vi "MultiColumnListbox_UnColorRows.vi"(7 "Parent VI Reference":refnum<vi>, 8 "error in":errorcluster, 10 "Color Rows":u32(colorbox)=16448250, 11 "MCL Reference":refnum<vi>) -> (0 "error out":errorcluster)   [LabVIEW 2014, in "hse-ui.lvlib"]
doc: "Colors the rows of a MCLB in alternate colors. If <b>Parent VI Reference</b> is supplied, panel updates are deferred.\n\n____\nHAMPEL SOFTWARE ENGINEERING v0.7.0 (2018-07-16 18:12)"
uses:
  hse-ui.lvlib
  MulticolumnListControl__System.ctl
  <vilib>/Utility/miscctls.llb/LVRowAndColumnTypeDef.ctl
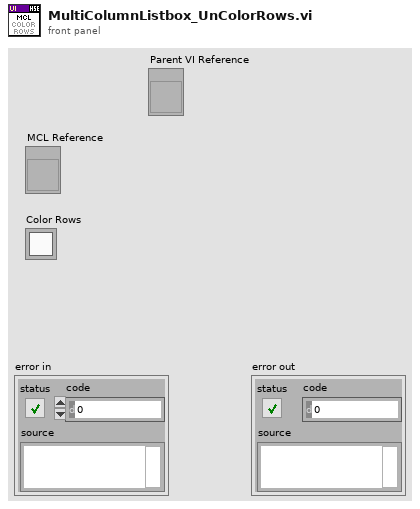
[diagram p1: front panel]
types:
  T1 = typedef "LVRowAndColumnTypeDef.ctl" = cluster{"Row":i32, "Column":i32}
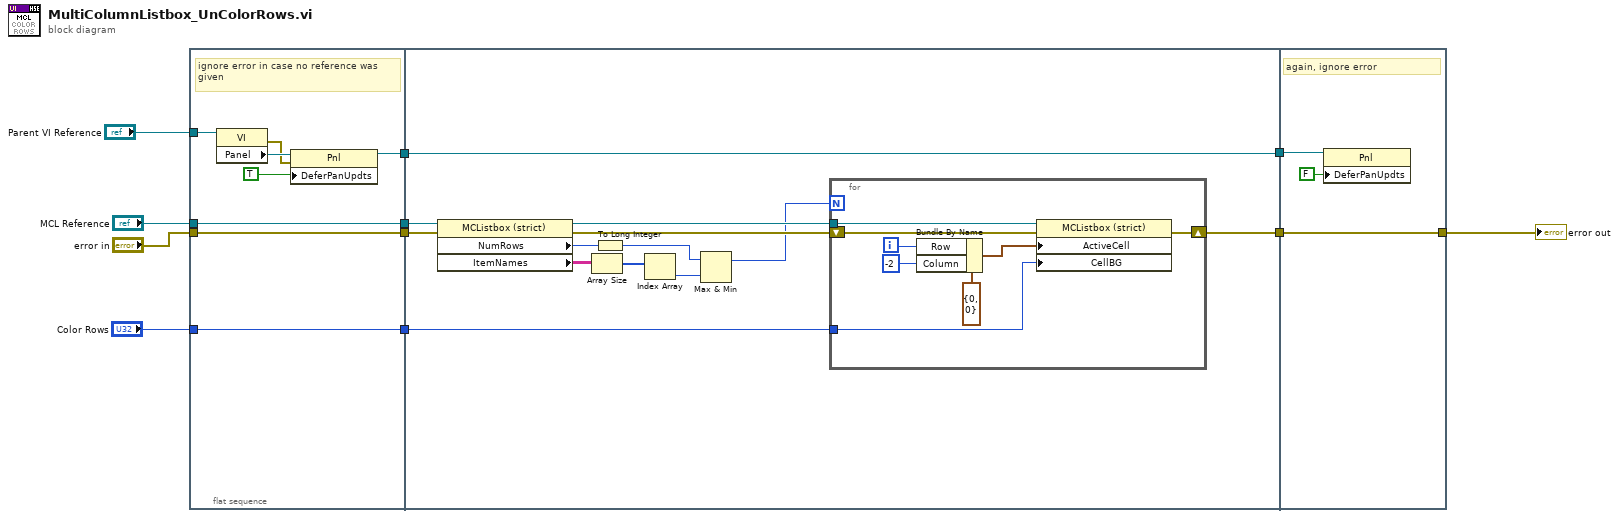
[diagram p0: block diagram]
diagram:
  n1 = flat-sequence {
    tunnel: "MCL Reference" -> [w19]
    tunnel: [w19] -> w10
    tunnel: [w15] -> w9
    tunnel: "error in" -> [w15]
    tunnel: "Parent VI Reference" -> [w14]
    tunnel: [w13] -> w6
    tunnel: "Color Rows" -> [w12]
    tunnel: [w12] -> w1
    tunnel: w10 -> [w26]
    tunnel: w9 -> [w24]
    tunnel: w6 -> [w23]
    tunnel: [w25] -> w5
    tunnel: [w23] -> w4
    tunnel: w1 -> [w21]
    tunnel: [w43] -> w3
    tunnel: w5 -> [w43]
    tunnel: w4 -> [w41]
    frame #0 {
      # "ignore error in case no reference was given"
      n2 = property class="VI"(reference=w14) -> (error out=w17:errorcluster, "Panel"=w18:refnum<vi>)  [unwired: 1 in, 1 out]
      n3 = property class="Pnl"(reference=w18, error in=w17, "DeferPanUpdts"=TRUE ("Defer Panel Updates")) -> (reference out=w13:refnum<vi>)  [unwired: 1 out]
    }
    frame #1 {
      n4 = property on="Property Node" class="MCListbox (strict)"(reference=w26, error in=w24) -> (reference out=w28:refnum<vi>, error out=w27:errorcluster, "NumRows"=w29:u32, "ItemNames"=w30:string[][])
      n5 = Array Size(array=w30) -> (size(s)=w32:i32[])
      n6 = To Long Integer(number=w29) -> (32bit integer=w22:i32)
      n7 = Index Array(array=w32) -> (element=w31:i32)  [unwired: 1 in]
      n8 = Max & Min(x=w22, y=w31) -> (max(x,y)=w20:i32)  [unwired: 1 out]
      n9 = for {
        N: w20 -> [_]
        tunnel: w28 -> [w40]
        tunnel: w21 -> [w34]
        shift-right: [w38] -> w25
        shift-left: w27 -> [w39]
        i -> [w33]
        n10 = Bundle By Name(cluster=T1 {"Row"=0, "Column"=0} ("Active Cell:Active Cell"), "Row"=w33, "Column"=-2) -> (w36:T1)
        n11 = property on="Property Node" class="MCListbox (strict)"(reference=w40, error in=w39, "ActiveCell"=w36, "CellBG"=w34) -> (error out=w38:errorcluster)  [unwired: 1 out]
      }
    }
    frame #2 {
      # "again, ignore error"
      n12 = property class="Pnl"(reference=w41, "DeferPanUpdts"=FALSE ("Defer Panel Updates")) -> ()  [unwired: 1 in, 2 out]
    }
  }
  "error out" <- w3
